vi "SIM_ysi.vi"(7 "Initialize":bool, 10 "Time Out (secs)":i32, 11 "YSI Com Port":i32) -> (0 "pH":dbl format="%.2f", 1 "Temperature":dbl format="%.2f", 2 "dis O2":dbl format="%.2f", 3 "ORP":dbl format="%.2f", 4 "spec K":dbl format="%.2f", 5 "Fresh Data":bool, 6 "Time out occurred":bool)   [LabVIEW 2016]
panel:
  in  "loop(ms)":u32=500
  in  "sim_ORP_high":dbl=200.0 format="%.2f"
  in  "sim_ORP_low":dbl=180.0 format="%.2f"
  in  "sim_pH_high":dbl=5.5 format="%.2f"
  in  "sim_pH_low":dbl=5.1 format="%.2f"
  in  "sim_dis_O2_high":dbl=7.0 format="%.2f"
  in  "sim_dis_O2_low":dbl=6.5 format="%.2f"
  in  "sim_spec_K_high":dbl=2000.0 format="%.2f"
  in  "sim_spec_K_low":dbl=1900.0 format="%.2f"
  in  "sim_temperature_high":dbl=15.0 format="%.2f"
  in  "sim_temperature_low":dbl=10.0 format="%.2f"
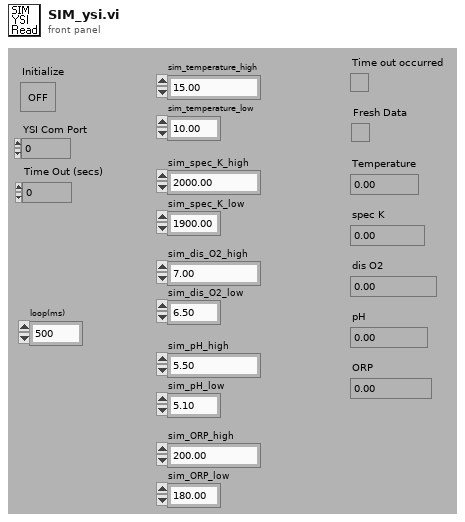
[diagram p1: front panel]
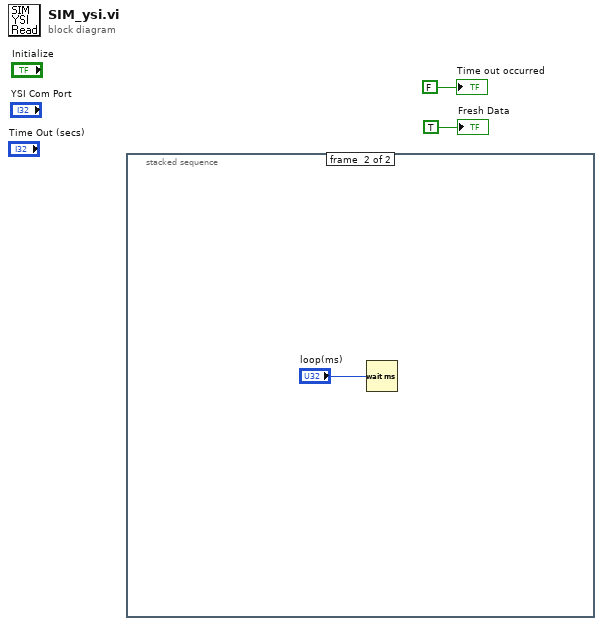
[diagram p0: block diagram]
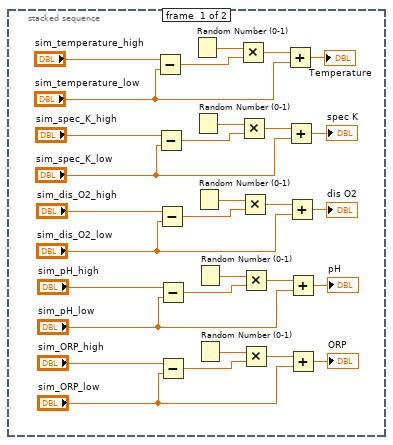
[diagram p2: hidden frame]
diagram:
  n1 = stacked-sequence {
    frame #0 {
      n2 = Subtract(x="sim_temperature_high", y="sim_temperature_low") -> (x-y=w30:dbl)
      n3 = Subtract(x="sim_spec_K_high", y="sim_spec_K_low") -> (x-y=w25:dbl)
      n4 = Subtract(x="sim_dis_O2_high", y="sim_dis_O2_low") -> (x-y=w20:dbl)
      n5 = Subtract(x="sim_pH_high", y="sim_pH_low") -> (x-y=w15:dbl)
      n6 = Subtract(x="sim_ORP_high", y="sim_ORP_low") -> (x-y=w10:dbl)
      n7 = Random Number (0-1)() -> (number: 0 to 1=w31:dbl)
      n8 = Random Number (0-1)() -> (number: 0 to 1=w26:dbl)
      n9 = Random Number (0-1)() -> (number: 0 to 1=w21:dbl)
      n10 = Random Number (0-1)() -> (number: 0 to 1=w16:dbl)
      n11 = Random Number (0-1)() -> (number: 0 to 1=w11:dbl)
      n12 = Multiply(x=w31, y=w30) -> (x*y=w29:dbl)
      n13 = Multiply(x=w26, y=w25) -> (x*y=w24:dbl)
      n14 = Multiply(x=w21, y=w20) -> (x*y=w19:dbl)
      n15 = Multiply(x=w16, y=w15) -> (x*y=w14:dbl)
      n16 = Multiply(x=w11, y=w10) -> (x*y=w9:dbl)
      n17 = Add(x=w29, y="sim_temperature_low") -> (x+y=→"Temperature":dbl)
      n18 = Add(x=w24, y="sim_spec_K_low") -> (x+y=→"spec K":dbl)
      n19 = Add(x=w19, y="sim_dis_O2_low") -> (x+y=→"dis O2":dbl)
      n20 = Add(x=w14, y="sim_pH_low") -> (x+y=→"pH":dbl)
      n21 = Add(x=w9, y="sim_ORP_low") -> (x+y=→"ORP":dbl)
    }
    frame #1 {
      n22 = Wait (ms)(milliseconds to wait="loop(ms)") -> ()  [unwired: 1 out]
    }
  }
  "Fresh Data" <- TRUE ("Fresh Data")
  "Time out occurred" <- FALSE ("Time out occurred")
